vi "treeTraverseComponentPropertiesRecursive.vi"(8 "error in (no error)":errorcluster, 9 "Indent (0)":i32, 10 "IPropertyObject in":refnum<class "IPropertyObject.lvclass">, 11 "Context in":T1) -> (0 "error out":errorcluster, 2 "IPropertyObject out":refnum<class "IPropertyObject.lvclass">, 3 "Context out":T1)   [LabVIEW 2022 SP3, in "Property Editor.lvlib"]
uses:
  <instrlib>/openDAQ/Examples/Property Editor/Property Editor.lvlib
  <instrlib>/openDAQ/Public/Classes/IPropertyObject/IPropertyObject.lvclass
  C:/Program Files (x86)/National Instruments/LabVIEW 2022/instr.lib/openDAQ/Public/Classes/IBaseObject/IBaseObject.lvclass
  <instrlib>/openDAQ/Examples/Property Editor/TypeDef/Context.ctl
  <instrlib>/openDAQ/Public/Classes/IComponent/IComponent.lvclass
  <instrlib>/openDAQ/Public/Classes/IProperty/IProperty.lvclass
  <instrlib>/openDAQ/Examples/Property Editor/TypeDef/DisplayType.ctl
  <instrlib>/openDAQ/Public/Classes/IBaseObject/IBaseObject.lvclass/IBaseObject.ctl
  <instrlib>/openDAQ/Public/Classes/IBaseObject/Accessor/Read reference.vi
  <instrlib>/openDAQ/Public/Classes/IBaseObject/Polymorphic/borrowInterface/borrowPropertyObjectInterface.vi
  <instrlib>/openDAQ/Public/Classes/IBaseObject/Polymorphic/borrowInterface/borrowListInterface.vi
  <instrlib>/openDAQ/Public/Classes/daqCoreTypes/IList/Polymorphic/getList/getStringList.vi
  <instrlib>/openDAQ/Public/Classes/daqCoreTypes/IList/Polymorphic/getList/getFloatList.vi
  <instrlib>/openDAQ/Public/Classes/IBaseObject/Polymorphic/borrowInterface/borrowDictInterface.vi
  <instrlib>/openDAQ/Public/Classes/daqCoreTypes/IDict/Polymorphic/getValueList/getBooleanValueList.vi
  <instrlib>/openDAQ/Public/Classes/daqCoreTypes/IDict/Polymorphic/getKeyList/getStringKeyList.vi
  <instrlib>/openDAQ/Public/Classes/daqCoreTypes/IDict/Polymorphic/getValueList/getIntegerValueList.vi
  <instrlib>/openDAQ/Public/Classes/daqCoreTypes/IDict/Polymorphic/getKeyList/getIntKeyList.vi
  <instrlib>/openDAQ/Public/Classes/IUnit/IUnit.lvclass
  <instrlib>/openDAQ/Public/Classes/IBaseObject/IBaseObject.lvclass
  <instrlib>/openDAQ/Public/Classes/daqCoreTypes/IList/IList.lvclass
  <instrlib>/openDAQ/Public/Classes/daqCoreTypes/IDict/IDict.lvclass
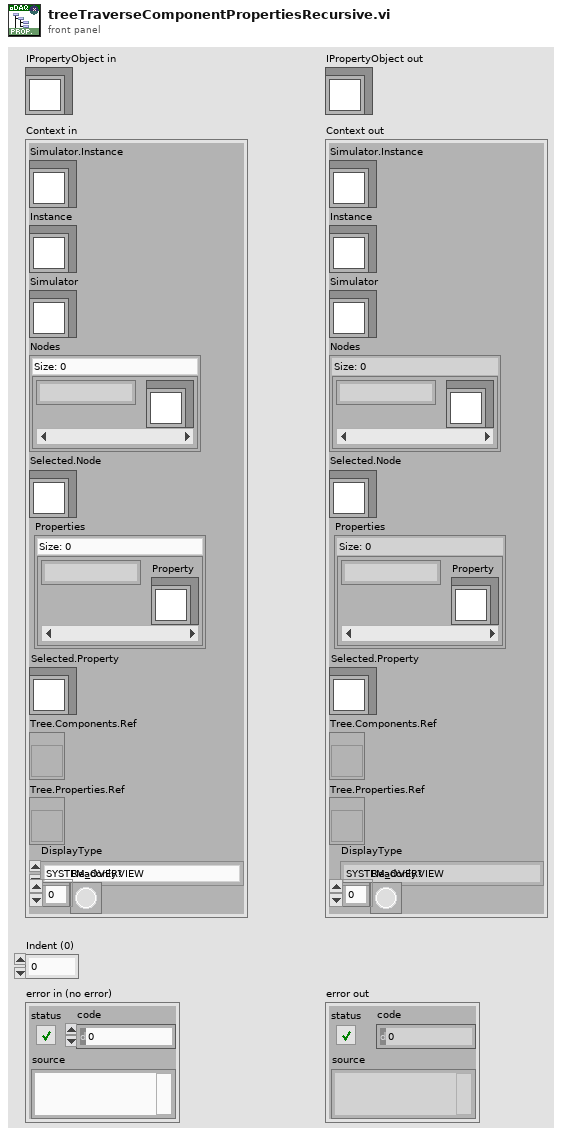
[diagram p1: front panel]
types:
  T1 = typedef "Property Editor.lvlib/Context.ctl" = cluster{"Simulator.Instance":refnum<class "IComponent.lvclass">, "Instance":refnum<class "IComponent.lvclass">, "Simulator":refnum<class "IComponent.lvclass">, "Nodes":map{string, refnum<class "IComponent.lvclass">}, "Selected.Node":refnum<class "IComponent.lvclass">, "Properties":map{string, refnum<class "IProperty.lvclass">}, "Selected.Property":refnum<class "IProperty.lvclass">, "Tree.Components.Ref":refnum<vi>, "Tree.Properties.Ref":refnum<vi>, "DisplayType":T2, "Readonly?":bool[]}
  T2 = typedef "Property Editor.lvlib/DisplayType.ctl" = enum16{"SYSTEM_OVERVIEW", "SIGNALS", "CHANNELS", "FUNCTION_BLOCKS", "TOPOLOGY", "TOPOLOGY_CUSTOM_COMPONENTS", "UNSPECIFIED"}
  T3 = typedef "openDAQ.lvlib/PropertyType.ctl" = u16
  T4 = typedef "openDAQ.lvlib/CoreType.ctl" = u16
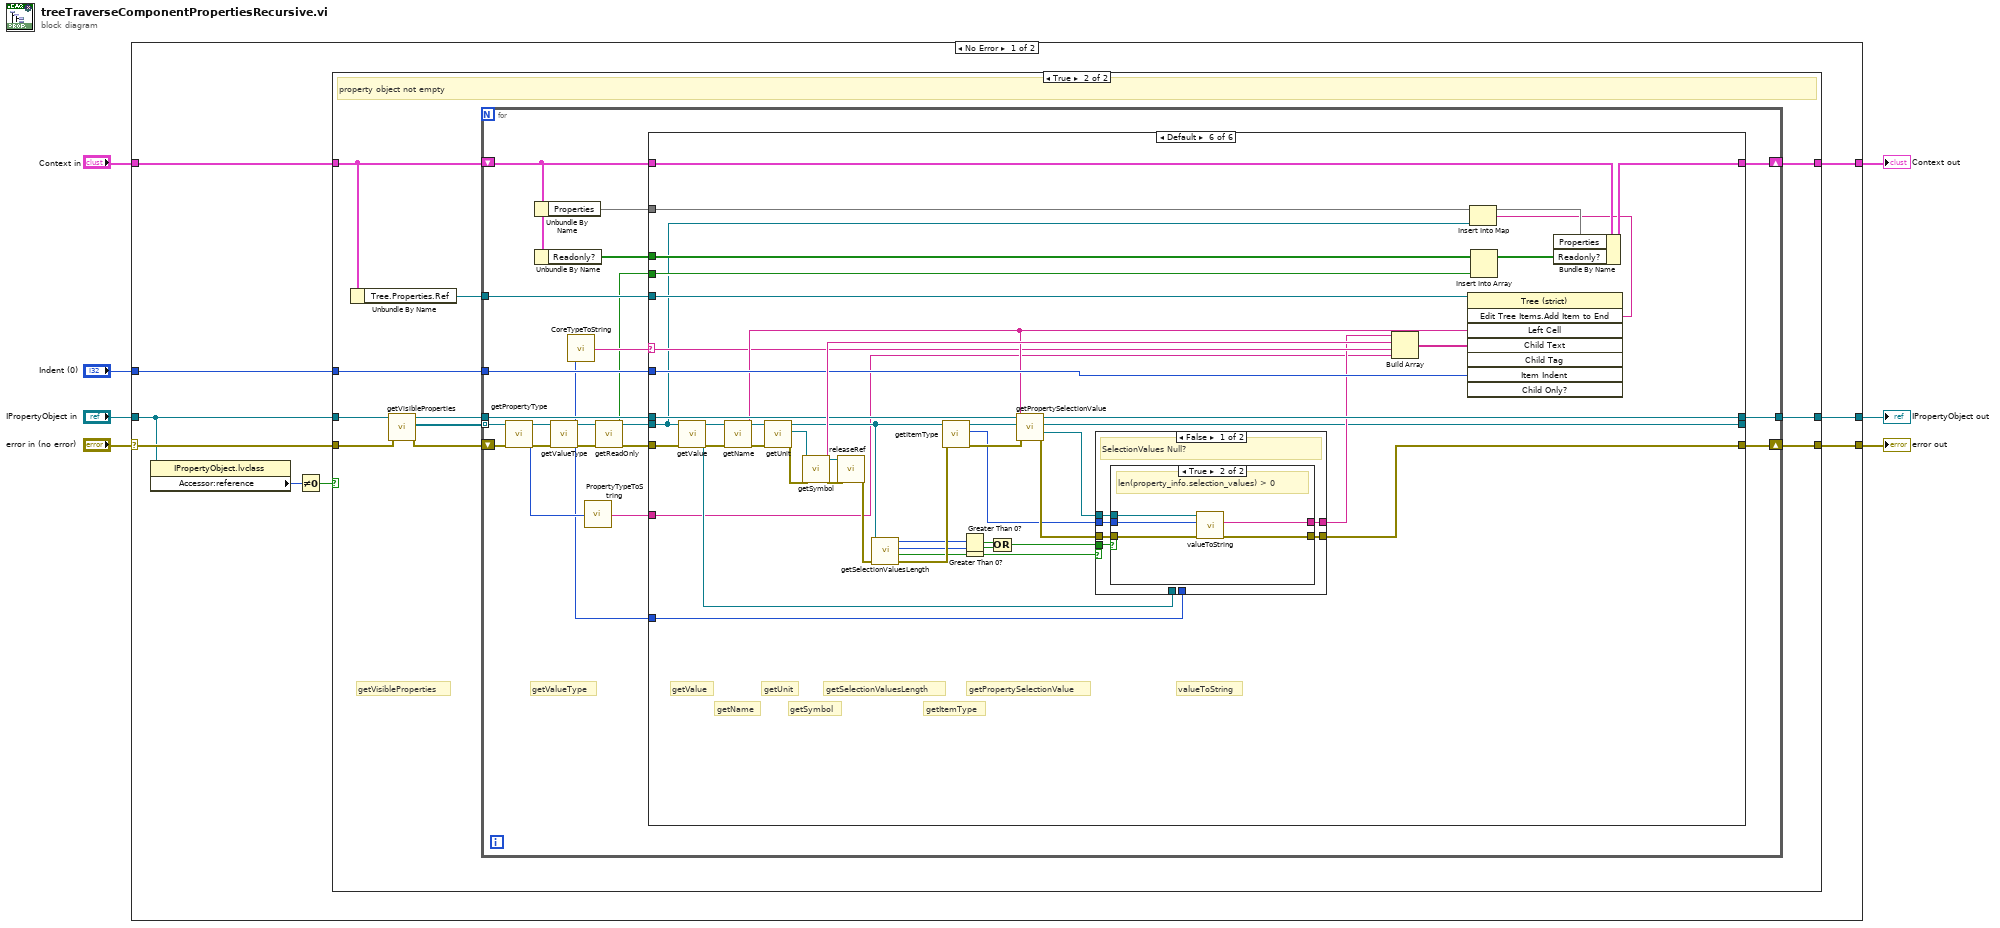
[diagram p0: block diagram]
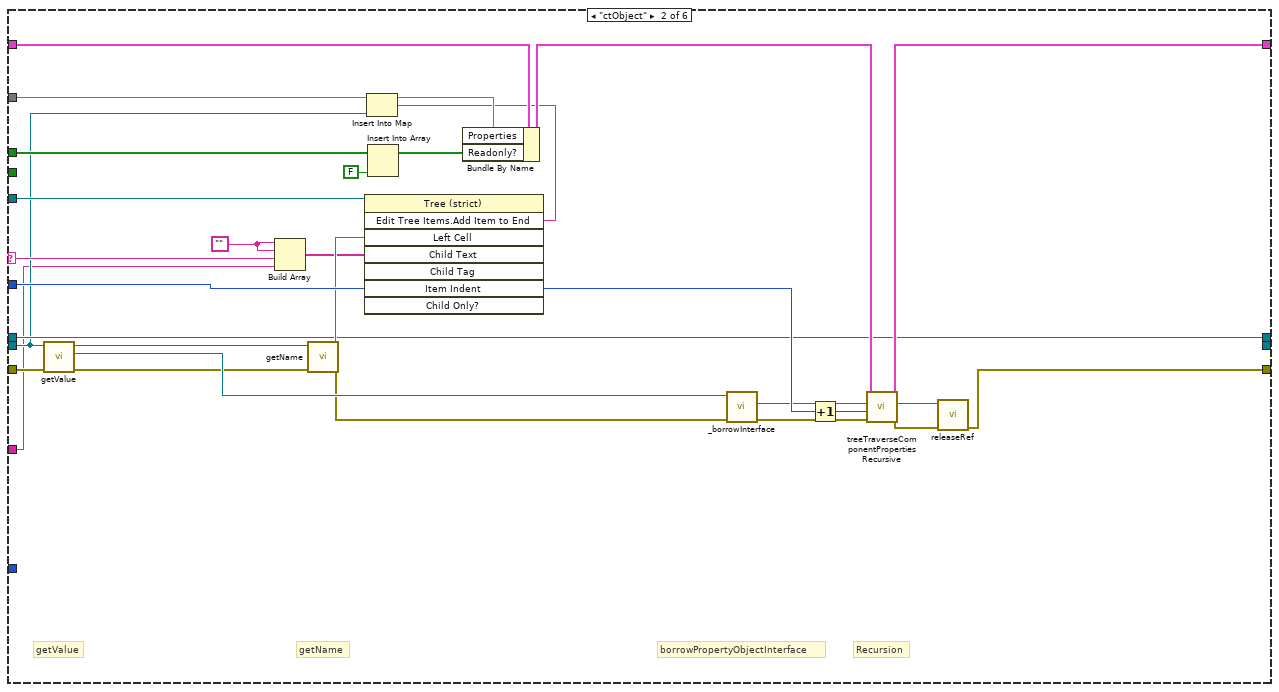
[diagram p4: hidden frame]
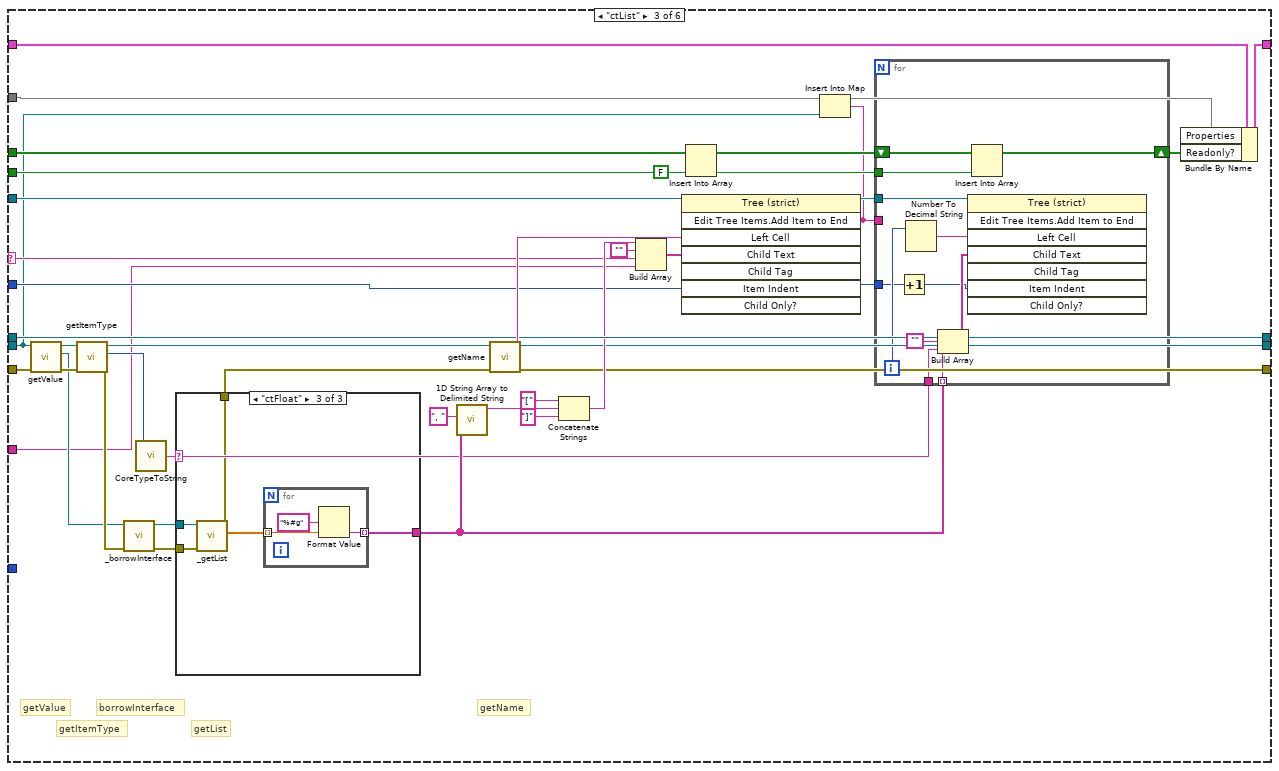
[diagram p5: hidden frame]
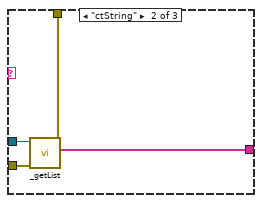
[diagram p7: hidden frame]
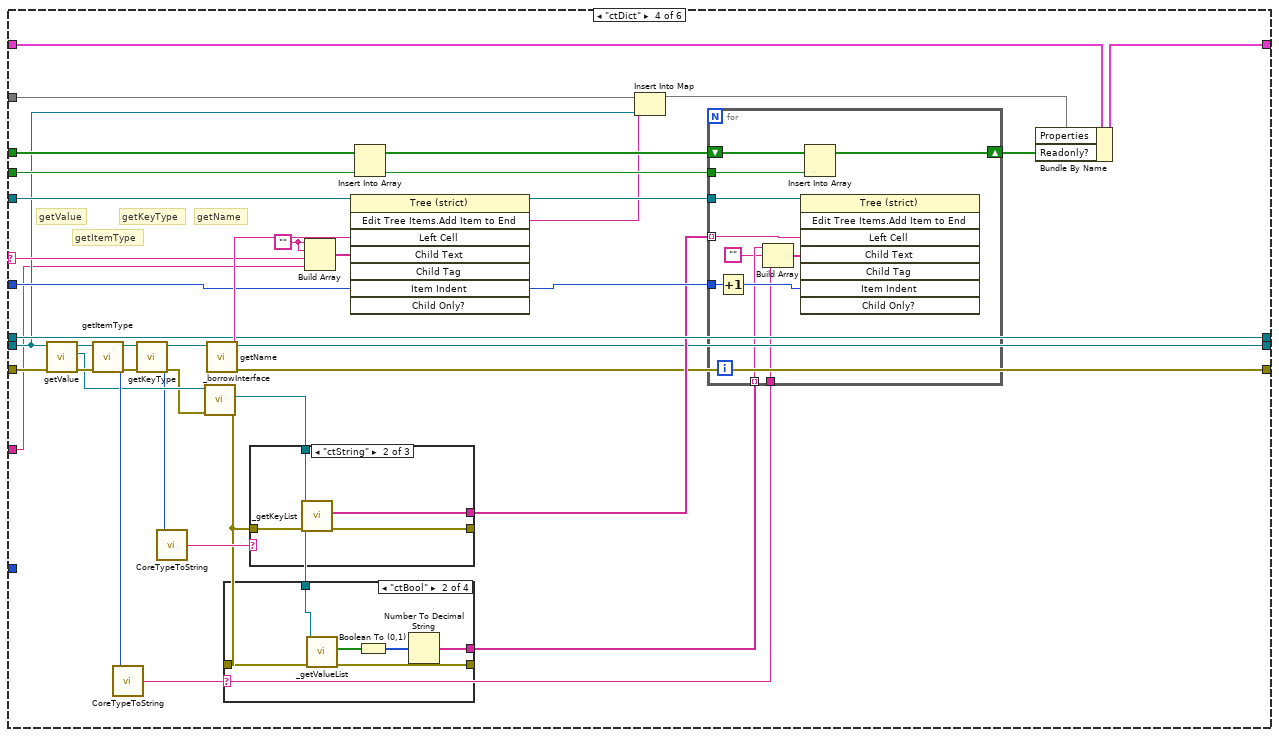
[diagram p8: hidden frame]
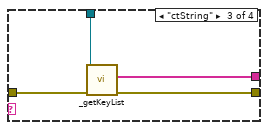
[diagram p10: hidden frame]
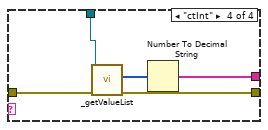
[diagram p11: hidden frame]
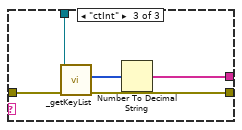
[diagram p13: hidden frame]
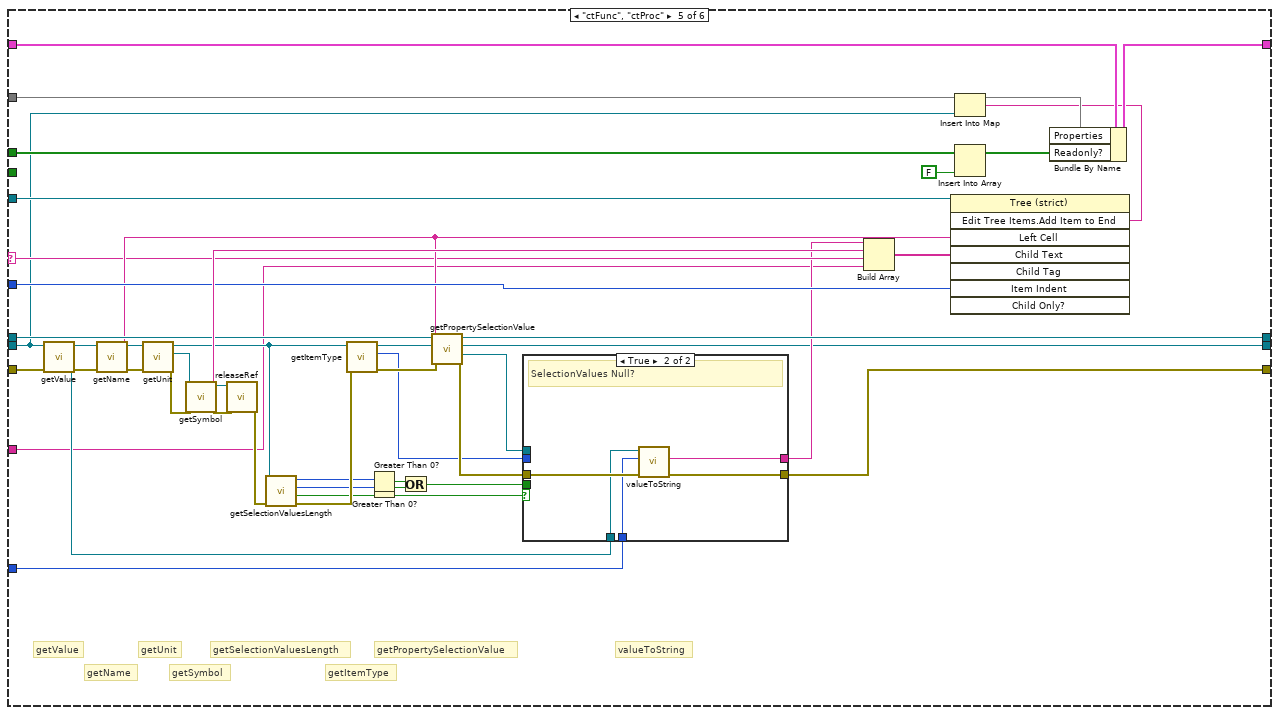
[diagram p14: hidden frame]
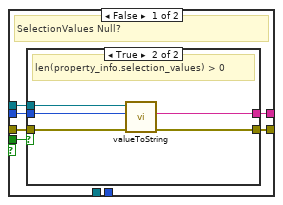
[diagram p15: hidden frame]
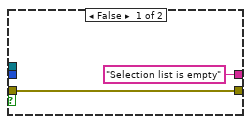
[diagram p16: hidden frame]
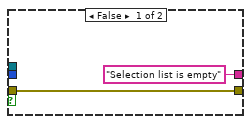
[diagram p17: hidden frame]
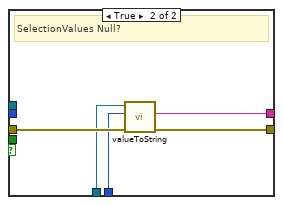
[diagram p18: hidden frame]
diagram:
  n1 = case shown="No Error" "error in (no error)" {
    selector: "error in (no error)" -> [w14 w352]
    tunnel: "IPropertyObject in" -> [w10 w351]
    tunnel: "Indent (0)" -> [w16 _]
    tunnel: [w15 w352] -> w5
    tunnel: [w13 w351] -> w3
    tunnel: "Context in" -> [w11 w350]
    tunnel: [w12 w350] -> w1
    frame No Error {
      n2 = property class="IPropertyObject.lvclass"(reference=w10) -> ("Accessor:reference"=w9:i64)  [unwired: 1 in, 2 out]
      n3 = Not Equal To 0?(x=w9) -> (x != 0?=w8:bool)
      n4 = case shown="True" w8 {
        tunnel: w10 -> [w19 w30]
        tunnel: w16 -> [_ w29]
        tunnel: [w18 w26] -> w15
        tunnel: w14 -> [w18 w25]
        tunnel: [w19 w23] -> w13
        tunnel: [w17 w22] -> w12
        tunnel: w11 -> [w17 w21]
        frame False {
          # "porperty object empty"
        }
        frame True {
          # "getVisibleProperties"
          # "property object not empty"
          n5 = Unbundle By Name(w21) -> ("Tree.Properties.Ref"=w20:refnum<vi>)
          n6 = call <instrlib>:"getVisibleProperties.vi"("error in (no error)"=w25, "IPropertyObject in"=w30) -> ("error out"=w28:errorcluster, "All Properties out"=w27:refnum<class "IProperty.lvclass">[], "IPropertyObject out"=w24:refnum<class "IPropertyObject.lvclass">)  [unwired: 7 in]
          n7 = for {
            tunnel: w27 -> [w34] mode=indexing
            tunnel: w20 -> [w52]
            tunnel: w29 -> [w50]
            shift-right: [w43] -> w26
            shift-left: w28 -> [w33]
            tunnel: w24 -> [w49]
            tunnel: [w48] -> w23
            shift-right: [w40] -> w22
            shift-left: w21 -> [w39]
            # "getValueType"
            n8 = call <instrlib>:"getPropertyType.vi"("error in (no error)"=w33, "IProperty in"=w34) -> ("error out"=w32:errorcluster, "Property Type out"=w37:T3, "IProperty out"=w31:refnum<class "IProperty.lvclass">)  [unwired: 7 in]
            n9 = Unbundle By Name(w39) -> ("Properties"=w38:map{string, refnum<class "IProperty.lvclass">})
            n10 = Unbundle By Name(w39) -> ("Readonly?"=w41:bool[])
            n11 = call <instrlib>:"getValueType.vi"("error in (no error)"=w32, "IProperty in"=w31) -> ("error out"=w46:errorcluster, "Value Type out"=w35:T4, "IProperty out"=w47:refnum<class "IProperty.lvclass">)  [unwired: 7 in]
            n12 = call <instrlib>:"CoreTypeToString.vi"("Value Type out"=w35) -> ("String"=w51:string)  [unwired: 4 in]
            n13 = call <instrlib>:"PropertyTypeToString.vi"("Property Type"=w37) -> ("String"=w36:string)  [unwired: 4 in]
            n14 = call <instrlib>:"getReadOnly.vi"("error in (no error)"=w46, "IProperty in"=w47) -> ("error out"=w44:errorcluster, "Read Only?"=w42:bool, "IProperty out"=w45:refnum<class "IProperty.lvclass">)  [unwired: 6 in, 1 out]
            n15 = case shown="Default" w51 {
              selector: w51 -> [_ w79 w103 w172 w237 w300]
              tunnel: [w56 w66 w99 w161 w234 w297] -> w43
              tunnel: w50 -> [_ w76 w105 w177 w255 w318]
              tunnel: w52 -> [_ w73 w120 w183 w254 w317]
              tunnel: w45 -> [w53 w59 w88 w152 w225 w288]
              tunnel: w44 -> [w56 w80 w123 w186 w264 w327]
              tunnel: w49 -> [w55 w72 w119 w182 w253 w316]
              tunnel: [w55 w72 w119 w182 w252 w315] -> w48
              tunnel: w35 -> [_ _ _ _ w239 w302]
              tunnel: w39 -> [w54 w65 w94 w156 w230 w293]
              tunnel: [w53 _ w98 w162 w235 w298] -> _
              tunnel: w41 -> [_ w69 w97 w160 w233 w296]
              tunnel: w42 -> [_ _ w91 w158 _ w295]
              tunnel: [w54 w85 w93 w155 w229 w292] -> w40
              tunnel: w38 -> [_ w62 w89 w154 w228 w291]
              tunnel: w36 -> [_ w57 w86 w150 w224 w287]
              frame "ctUndefined" {
              }
              frame "ctObject" {
                w71 = ""
                # "Recursion"
                # "getName"
                # "borrowPropertyObjectInterface"
                # "getValue"
                n16 = call <instrlib>:"getValue.vi"("error in (no error)"=w80, "IProperty in"=w59) -> ("error out"=w81:errorcluster, "Value out"=w82:refnum<class "IBaseObject.lvclass">, "IProperty out"=w83:refnum<class "IProperty.lvclass">)  [unwired: 7 in]
                n17 = Build Array(w71, w71, w79, w57) -> (w74:string[])
                n18 = call <instrlib>:"getName.vi"("error in (no error)"=w81, "IProperty in"=w83) -> ("error out"=w58:errorcluster, "Name out"=w75:string)  [unwired: 7 in, 1 out]
                n19 = invoke class="Tree (strict)" method="Edit Tree Items.Add Item to End"(reference=w73, "Left Cell"=w75, "Child Text"=w74, "Item Indent"=w76) -> ("Edit Tree Items:Add Item to End"=w60:string)  [unwired: 4 in, 7 out]
                n20 = Insert Into Map(map in=w62, key=w60, value=w59) -> (map out=w61:map{string, refnum<class "IProperty.lvclass">})  [unwired: 2 out]
                n21 = Insert Into Array(array=w69, new element=FALSE ("new element/subarray")) -> (w64:bool[])  [unwired: 1 in]
                n22 = Bundle By Name(cluster=w65, "Properties"=w61, "Readonly?"=w64) -> (w84:T1)
                n23 = call-poly <instrlib>:"_borrowInterface.vi"("error in (no error)"=w58, "IBaseObject in"=w82) -> ("error out"=w78:errorcluster, "PropertyObject out"=w70:refnum<class "IPropertyObject.lvclass">)  [unwired: 6 in, 2 out]
                n24 = Increment(x=w76) -> (x+1=w77:i32)
                n25 = call <instrlib>:"treeTraverseComponentPropertiesRecursive.vi"("error in (no error)"=w78, "Indent (0)"=w77, "IPropertyObject in"=w70, "Context in"=w84) -> ("error out"=w67:errorcluster, "IPropertyObject out"=w68:refnum<class "IPropertyObject.lvclass">, "Context out"=w85:T1)  [unwired: 5 in]
                n26 = call-dynamic "releaseRef.vi"("error in (no error)"=w67, "IBaseObject in"=w68) -> ("error out"=w66:errorcluster)  [unwired: 9 in]
              }
              frame "ctList" {
                # "getList"
                # "borrowInterface"
                # "getItemType"
                # "getName"
                # "getValue"
                n27 = call <instrlib>:"getValue.vi"("error in (no error)"=w123, "IProperty in"=w88) -> ("error out"=w116:errorcluster, "Value out"=w114:refnum<class "IBaseObject.lvclass">, "IProperty out"=w117:refnum<class "IProperty.lvclass">)  [unwired: 7 in]
                n28 = call <instrlib>:"getItemType.vi"("error in (no error)"=w116, "IProperty in"=w117) -> ("error out"=w124:errorcluster, "Item Type out"=w115:T4, "IProperty out"=w118:refnum<class "IProperty.lvclass">)  [unwired: 7 in]
                n29 = call-poly <instrlib>:"_borrowInterface.vi"("error in (no error)"=w124, "IBaseObject in"=w114) -> ("error out"=w102:errorcluster, "List out"=w101:refnum<class "IList.lvclass">)  [unwired: 6 in, 2 out]
                n30 = call <instrlib>:"CoreTypeToString.vi"("Value Type out"=w115) -> ("String"=w104:string)  [unwired: 4 in]
                n31 = case shown="\"ctFloat\"" w104 {
                  tunnel: [w137 w141 w146] -> w113
                  tunnel: [_ w140 w144] -> w112
                  tunnel: w102 -> [w137 w139 w143]
                  tunnel: w101 -> [_ w138 w142]
                  frame Default {
                  }
                  frame "ctString" {
                    n32 = call-poly <instrlib>:"_getList.vi"("error in (no error)"=w139, "IList in"=w138) -> ("error out"=w141:errorcluster, "String List out"=w140:string[])  [unwired: 8 in]
                  }
                  frame "ctFloat" {
                    n33 = call-poly <instrlib>:"_getList.vi"("error in (no error)"=w143, "IList in"=w142) -> ("error out"=w146:errorcluster, "Floats out"=w145:dbl[])  [unwired: 8 in]
                    n34 = for {
                      tunnel: w145 -> [w149] mode=indexing
                      tunnel: [w148] -> w144 mode=indexing
                      n35 = Format Value(format string="%#g", value (0)=w149) -> (output string=w148:string)  [unwired: 1 in]
                    }
                  }
                }
                n36 = call <vilib>:"1D String Array to Delimited String.vi"("delimiter"=", ", "string array"=w112) -> ("delimited string"=w108:string)  [unwired: 9 in]
                n37 = call <instrlib>:"getName.vi"("error in (no error)"=w113, "IProperty in"=w118) -> ("error out"=w99:errorcluster, "Name out"=w122:string, "IProperty out"=w98:refnum<class "IProperty.lvclass">)  [unwired: 7 in]
                n38 = Concatenate Strings("[", w108, "]") -> (w109:string)
                n39 = Build Array(w109, "" ("element"), w103, w86) -> (w121:string[])
                n40 = invoke class="Tree (strict)" method="Edit Tree Items.Add Item to End"(reference=w120, "Left Cell"=w122, "Child Text"=w121, "Item Indent"=w105) -> (reference out=w100:refnum<vi>, "Edit Tree Items:Add Item to End"=w90:string)  [unwired: 4 in, 6 out]
                n41 = Insert Into Array(array=w97, new element=FALSE ("new element/subarray")) -> (w96:bool[])  [unwired: 1 in]
                n42 = Insert Into Map(map in=w89, key=w90, value=w88) -> (map out=w87:map{string, refnum<class "IProperty.lvclass">})  [unwired: 2 out]
                n43 = for {
                  tunnel: w112 -> [w136] mode=indexing
                  tunnel: w105 -> [w132]
                  tunnel: w104 -> [w129]
                  tunnel: w100 -> [w128]
                  shift-right: [w126] -> w95
                  shift-left: w96 -> [w127]
                  tunnel: w91 -> [w125]
                  tunnel: w90 -> [_]
                  i -> [w134]
                  n44 = Increment(x=w132) -> (x+1=w131:i32)
                  n45 = Number To Decimal String(number=w134) -> (decimal integer string=w133:string)  [unwired: 1 in]
                  n46 = Build Array(w136, "" ("element"), w129) -> (w135:string[])
                  n47 = invoke class="Tree (strict)" method="Edit Tree Items.Add Item to End"(reference=w128, "Left Cell"=w133, "Child Text"=w135, "Item Indent"=w131) -> ()  [unwired: 4 in, 8 out]
                  n48 = Insert Into Array(array=w127, new element=w125) -> (w126:bool[])  [unwired: 1 in]
                }
                n49 = Bundle By Name(cluster=w94, "Properties"=w87, "Readonly?"=w95) -> (w93:T1)
              }
              frame "ctDict" {
                w171 = "" ("element")
                # "getKeyType"
                # "getItemType"
                # "getName"
                # "getValue"
                n50 = call <instrlib>:"getValue.vi"("error in (no error)"=w186, "IProperty in"=w152) -> ("error out"=w180:errorcluster, "Value out"=w178:refnum<class "IBaseObject.lvclass">, "IProperty out"=w181:refnum<class "IProperty.lvclass">)  [unwired: 7 in]
                n51 = call <instrlib>:"getItemType.vi"("error in (no error)"=w180, "IProperty in"=w181) -> ("error out"=w174:errorcluster, "Item Type out"=w179:T4, "IProperty out"=w176:refnum<class "IProperty.lvclass">)  [unwired: 7 in]
                n52 = call <instrlib>:"CoreTypeToString.vi"("Value Type out"=w179) -> ("String"=w164:string)  [unwired: 4 in]
                n53 = call <instrlib>:"getKeyType.vi"("error in (no error)"=w174, "IProperty in"=w176) -> ("error out"=w170:errorcluster, "Key Type out"=w173:T4, "IProperty out"=w175:refnum<class "IProperty.lvclass">)  [unwired: 7 in]
                n54 = call <instrlib>:"CoreTypeToString.vi"("Value Type out"=w173) -> ("String"=w169:string)  [unwired: 4 in]
                n55 = call-poly <instrlib>:"_borrowInterface.vi"("error in (no error)"=w170, "IBaseObject in"=w178) -> ("error out"=w167:errorcluster, "Dict out"=w168:refnum<class "IDict.lvclass">)  [unwired: 6 in, 2 out]
                n56 = call <instrlib>:"getName.vi"("IProperty in"=w175) -> ("error out"=w161:errorcluster, "Name out"=w185:string, "IProperty out"=w162:refnum<class "IProperty.lvclass">)  [unwired: 8 in]
                n57 = case shown="\"ctBool\"" w164 {
                  tunnel: w168 -> [_ w193 w197 w202]
                  tunnel: w167 -> [w187 w192 w196 w201]
                  tunnel: [_ w190 w195 w198] -> w165
                  tunnel: [w187 w191 w194 w200] -> _
                  frame Default {
                  }
                  frame "ctBool" {
                    n58 = call-poly <instrlib>:"_getValueList.vi"("error in (no error)"=w192, "IDict in"=w193) -> ("error out"=w191:errorcluster, "Boolean Value list out"=w189:bool[])  [unwired: 7 in, 1 out]
                    n59 = Boolean To (0,1)(Boolean=w189) -> (0, 1=w188:i16[])
                    n60 = Number To Decimal String(number=w188) -> (decimal integer string=w190:string[])  [unwired: 1 in]
                  }
                  frame "ctString" {
                    n61 = call-poly <instrlib>:"_getKeyList.vi"("error in (no error)"=w196, "IDict in"=w197) -> ("error out"=w194:errorcluster, "Key List out"=w195:string[])  [unwired: 7 in, 1 out]
                  }
                  frame "ctInt" {
                    n62 = call-poly <instrlib>:"_getValueList.vi"("error in (no error)"=w201, "IDict in"=w202) -> ("error out"=w200:errorcluster, "Integer Value list out"=w199:i32[])  [unwired: 7 in, 1 out]
                    n63 = Number To Decimal String(number=w199) -> (decimal integer string=w198:string[])  [unwired: 1 in]
                  }
                }
                n64 = case shown="\"ctString\"" w169 {
                  tunnel: w168 -> [_ w207 w212]
                  tunnel: w167 -> [w203 w206 w211]
                  tunnel: [_ w205 w208] -> w166
                  tunnel: [w203 w204 w210] -> _
                  frame Default {
                  }
                  frame "ctString" {
                    n65 = call-poly <instrlib>:"_getKeyList.vi"("error in (no error)"=w206, "IDict in"=w207) -> ("error out"=w204:errorcluster, "Key List out"=w205:string[])  [unwired: 7 in, 1 out]
                  }
                  frame "ctInt" {
                    n66 = call-poly <instrlib>:"_getKeyList.vi"("error in (no error)"=w211, "IDict in"=w212) -> ("error out"=w210:errorcluster, "Key List out"=w209:i32[])  [unwired: 7 in, 1 out]
                    n67 = Number To Decimal String(number=w209) -> (decimal integer string=w208:string[])  [unwired: 1 in]
                  }
                }
                n68 = Build Array(w171, w171, w172, w150) -> (w184:string[])
                n69 = invoke class="Tree (strict)" method="Edit Tree Items.Add Item to End"(reference=w183, "Left Cell"=w185, "Child Text"=w184, "Item Indent"=w177) -> (reference out=w163:refnum<vi>, "Edit Tree Items:Add Item to End"=w153:string)  [unwired: 4 in, 6 out]
                n70 = Insert Into Array(array=w160, new element=w158) -> (w159:bool[])  [unwired: 1 in]
                n71 = Insert Into Map(map in=w154, key=w153, value=w152) -> (map out=w151:map{string, refnum<class "IProperty.lvclass">})  [unwired: 2 out]
                n72 = for {
                  tunnel: w177 -> [w223]
                  tunnel: w166 -> [w221] mode=indexing
                  tunnel: w165 -> [w220] mode=indexing
                  tunnel: w164 -> [w218]
                  tunnel: w163 -> [w216]
                  shift-right: [w214] -> w157
                  shift-left: w159 -> [w215]
                  tunnel: w158 -> [w213]
                  n73 = Increment(x=w223) -> (x+1=w222:i32)
                  n74 = Build Array(w220, "" ("element"), w218) -> (w219:string[])
                  n75 = invoke class="Tree (strict)" method="Edit Tree Items.Add Item to End"(reference=w216, "Left Cell"=w221, "Child Text"=w219, "Item Indent"=w222) -> ()  [unwired: 4 in, 8 out]
                  n76 = Insert Into Array(array=w215, new element=w213) -> (w214:bool[])  [unwired: 1 in]
                }
                n77 = Bundle By Name(cluster=w156, "Properties"=w151, "Readonly?"=w157) -> (w155:T1)
              }
              frame "ctFunc", "ctProc" {
                # "valueToString"
                # "getSelectionValuesLength"
                # "getPropertySelectionValue"
                # "getItemType"
                # "getSymbol"
                # "getUnit"
                # "getName"
                # "getValue"
                n78 = call <instrlib>:"getValue.vi"("error in (no error)"=w264, "IProperty in"=w225) -> ("error out"=w265:errorcluster, "Value out"=w238:refnum<class "IBaseObject.lvclass">, "IProperty out"=w266:refnum<class "IProperty.lvclass">)  [unwired: 7 in]
                n79 = call <instrlib>:"getName.vi"("error in (no error)"=w265, "IProperty in"=w266) -> ("error out"=w257:errorcluster, "Name out"=w250:string, "IProperty out"=w258:refnum<class "IProperty.lvclass">)  [unwired: 7 in]
                n80 = call <instrlib>:"getUnit.vi"("error in (no error)"=w257, "IProperty in"=w258) -> ("error out"=w262:errorcluster, "Unit out"=w263:refnum<class "IUnit.lvclass">, "IProperty out"=w247:refnum<class "IProperty.lvclass">)  [unwired: 7 in]
                n81 = call <instrlib>:"getSymbol.vi"("error in (no error)"=w262, "IUnit in"=w263) -> ("error out"=w260:errorcluster, "Symbol out"=w259:string, "IUnit out"=w261:refnum<class "IUnit.lvclass">)  [unwired: 7 in]
                n82 = call-dynamic "releaseRef.vi"("error in (no error)"=w260, "IBaseObject in"=w261) -> ("error out"=w246:errorcluster)  [unwired: 9 in]
                n83 = call <instrlib>:"getSelectionValuesLength.vi"("error in (no error)"=w246, "IProperty in"=w247) -> ("error out"=w267:errorcluster, "Selection Values Null?"=w245:bool, "List.Size"=w243:i32, "Dict.Size"=w244:i32)  [unwired: 4 in, 2 out]
                n84 = call <instrlib>:"getItemType.vi"("error in (no error)"=w267, "IProperty in"=w247) -> ("error out"=w251:errorcluster, "Item Type out"=w249:T4, "IProperty out"=w235:refnum<class "IProperty.lvclass">)  [unwired: 7 in]
                n85 = Greater Than 0?(x=w244) -> (x > 0?=w242:bool)
                n86 = Greater Than 0?(x=w243) -> (x > 0?=w241:bool)
                n87 = Or(x=w242, y=w241) -> (x .or. y?=w240:bool)
                n88 = call <instrlib>:"getPropertySelectionValue.vi"("error in (no error)"=w251, "Property Name in"=w250, "IPropertyObject in"=w253) -> ("error out"=w268:errorcluster, "Property Selection Value out"=w248:refnum<class "IBaseObject.lvclass">, "IPropertyObject out"=w252:refnum<class "IPropertyObject.lvclass">)  [unwired: 5 in, 1 out]
                n89 = case shown="True" w245 {
                  tunnel: [w271 w285] -> w234
                  tunnel: w249 -> [w273 _]
                  tunnel: w268 -> [w272 w286]
                  tunnel: w248 -> [w274 _]
                  tunnel: w240 -> [w269 _]
                  tunnel: [w270 w284] -> w236
                  tunnel: w239 -> [_ w283]
                  tunnel: w238 -> [_ w282]
                  frame False {
                    # "SelectionValues Null?"
                    n90 = case shown="True" w269 {
                      tunnel: w274 -> [_ w281]
                      tunnel: w273 -> [_ w280]
                      tunnel: w272 -> [w276 w279]
                      tunnel: [w276 w278] -> w271
                      tunnel: ["Selection list is empty" ("String out") w277] -> w270
                      frame False {
                      }
                      frame True {
                        # "len(property_info.selection_values) > 0"
                        n91 = call <instrlib>:"valueToString.vi"("error in (no error)"=w279, "Value Type in"=w280, "Value in"=w281) -> ("error out"=w278:errorcluster, "String out"=w277:string)  [unwired: 6 in, 1 out]
                      }
                    }
                  }
                  frame True {
                    # "SelectionValues Null?"
                    n92 = call <instrlib>:"valueToString.vi"("error in (no error)"=w286, "Value Type in"=w283, "Value in"=w282) -> ("error out"=w285:errorcluster, "String out"=w284:string)  [unwired: 6 in, 1 out]
                  }
                }
                n93 = Build Array(w236, w259, w237, w224) -> (w256:string[])
                n94 = invoke class="Tree (strict)" method="Edit Tree Items.Add Item to End"(reference=w254, "Left Cell"=w250, "Child Text"=w256, "Item Indent"=w255) -> ("Edit Tree Items:Add Item to End"=w226:string)  [unwired: 4 in, 7 out]
                n95 = Insert Into Map(map in=w228, key=w226, value=w225) -> (map out=w227:map{string, refnum<class "IProperty.lvclass">})  [unwired: 2 out]
                n96 = Insert Into Array(array=w233, new element=FALSE) -> (w231:bool[])  [unwired: 1 in]
                n97 = Bundle By Name(cluster=w230, "Properties"=w227, "Readonly?"=w231) -> (w229:T1)
              }
              frame Default {
                # "valueToString"
                # "getSelectionValuesLength"
                # "getPropertySelectionValue"
                # "getItemType"
                # "getSymbol"
                # "getUnit"
                # "getName"
                # "getValue"
                n98 = call <instrlib>:"getValue.vi"("error in (no error)"=w327, "IProperty in"=w288) -> ("error out"=w328:errorcluster, "Value out"=w301:refnum<class "IBaseObject.lvclass">, "IProperty out"=w329:refnum<class "IProperty.lvclass">)  [unwired: 7 in]
                n99 = call <instrlib>:"getName.vi"("error in (no error)"=w328, "IProperty in"=w329) -> ("error out"=w320:errorcluster, "Name out"=w313:string, "IProperty out"=w321:refnum<class "IProperty.lvclass">)  [unwired: 7 in]
                n100 = call <instrlib>:"getUnit.vi"("error in (no error)"=w320, "IProperty in"=w321) -> ("error out"=w325:errorcluster, "Unit out"=w326:refnum<class "IUnit.lvclass">, "IProperty out"=w310:refnum<class "IProperty.lvclass">)  [unwired: 7 in]
                n101 = call <instrlib>:"getSymbol.vi"("error in (no error)"=w325, "IUnit in"=w326) -> ("error out"=w323:errorcluster, "Symbol out"=w322:string, "IUnit out"=w324:refnum<class "IUnit.lvclass">)  [unwired: 7 in]
                n102 = call-dynamic "releaseRef.vi"("error in (no error)"=w323, "IBaseObject in"=w324) -> ("error out"=w309:errorcluster)  [unwired: 9 in]
                n103 = call <instrlib>:"getSelectionValuesLength.vi"("error in (no error)"=w309, "IProperty in"=w310) -> ("error out"=w330:errorcluster, "Selection Values Null?"=w308:bool, "List.Size"=w306:i32, "Dict.Size"=w307:i32)  [unwired: 4 in, 2 out]
                n104 = call <instrlib>:"getItemType.vi"("error in (no error)"=w330, "IProperty in"=w310) -> ("error out"=w314:errorcluster, "Item Type out"=w312:T4, "IProperty out"=w298:refnum<class "IProperty.lvclass">)  [unwired: 7 in]
                n105 = Greater Than 0?(x=w307) -> (x > 0?=w305:bool)
                n106 = Greater Than 0?(x=w306) -> (x > 0?=w304:bool)
                n107 = Or(x=w305, y=w304) -> (x .or. y?=w303:bool)
                n108 = call <instrlib>:"getPropertySelectionValue.vi"("error in (no error)"=w314, "Property Name in"=w313, "IPropertyObject in"=w316) -> ("error out"=w331:errorcluster, "Property Selection Value out"=w311:refnum<class "IBaseObject.lvclass">, "IPropertyObject out"=w315:refnum<class "IPropertyObject.lvclass">)  [unwired: 5 in, 1 out]
                n109 = case shown="False" w308 {
                  tunnel: [w334 w348] -> w297
                  tunnel: w312 -> [w336 _]
                  tunnel: w331 -> [w335 w349]
                  tunnel: w311 -> [w337 _]
                  tunnel: w303 -> [w332 _]
                  tunnel: [w333 w347] -> w299
                  tunnel: w302 -> [_ w346]
                  tunnel: w301 -> [_ w345]
                  frame False {
                    # "SelectionValues Null?"
                    n110 = case shown="True" w332 {
                      tunnel: w337 -> [_ w344]
                      tunnel: w336 -> [_ w343]
                      tunnel: w335 -> [w339 w342]
                      tunnel: [w339 w341] -> w334
                      tunnel: ["Selection list is empty" ("String out") w340] -> w333
                      frame False {
                      }
                      frame True {
                        # "len(property_info.selection_values) > 0"
                        n111 = call <instrlib>:"valueToString.vi"("error in (no error)"=w342, "Value Type in"=w343, "Value in"=w344) -> ("error out"=w341:errorcluster, "String out"=w340:string)  [unwired: 6 in, 1 out]
                      }
                    }
                  }
                  frame True {
                    # "SelectionValues Null?"
                    n112 = call <instrlib>:"valueToString.vi"("error in (no error)"=w349, "Value Type in"=w346, "Value in"=w345) -> ("error out"=w348:errorcluster, "String out"=w347:string)  [unwired: 6 in, 1 out]
                  }
                }
                n113 = Build Array(w299, w322, w300, w287) -> (w319:string[])
                n114 = invoke class="Tree (strict)" method="Edit Tree Items.Add Item to End"(reference=w317, "Left Cell"=w313, "Child Text"=w319, "Item Indent"=w318) -> ("Edit Tree Items:Add Item to End"=w289:string)  [unwired: 4 in, 7 out]
                n115 = Insert Into Map(map in=w291, key=w289, value=w288) -> (map out=w290:map{string, refnum<class "IProperty.lvclass">})  [unwired: 2 out]
                n116 = Insert Into Array(array=w296, new element=w295) -> (w294:bool[])  [unwired: 1 in]
                n117 = Bundle By Name(cluster=w293, "Properties"=w290, "Readonly?"=w294) -> (w292:T1)
              }
            }
          }
        }
      }
    }
    frame Error {
    }
  }
  "error out" <- w5
  "IPropertyObject out" <- w3
  "Context out" <- w1
